vi "StatsToPlugin.vi"() -> ()   [LabVIEW 2011]
panel:
  out "Plug in titles":string[](array[string])
  out "Plug in values":string[](array[string])
  in  "AdditionalNote":string
  in  "Stats":T1(array[cluster]) {"Min" format="%0.2f"; "Max" format="%0.2f"; "mean(5Maxs)" format="%0.2f"; "mean(5Mins)" format="%0.2f"; "SD(Cp)" format="%0.2f"; "meanCp" format="%0.2f"}
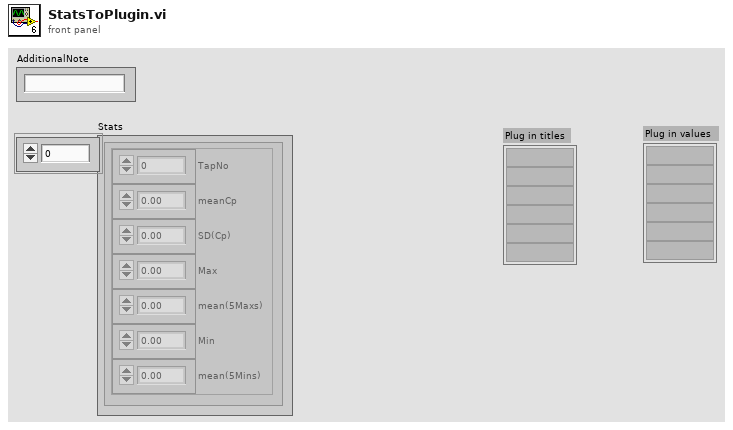
[diagram p1: front panel]
types:
  T1 = cluster{"TapNo":i32, "meanCp":dbl, "SD(Cp)":dbl, "Max":dbl, "mean(5Maxs)":dbl, "Min":dbl, "mean(5Mins)":dbl}[]
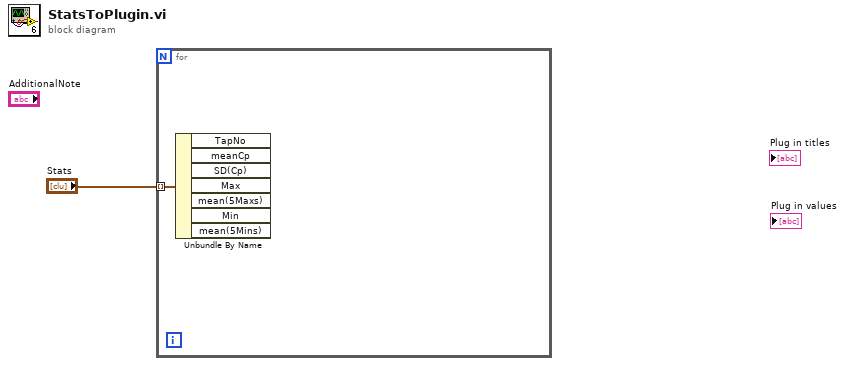
[diagram p0: block diagram]
diagram:
  n1 = for {
    tunnel: "Stats" -> [w2] mode=indexing
    n2 = Unbundle By Name(w2) -> ()  [unwired: 7 out]
  }
